vi "Get ChildNode by ctrl.vi"(8 "error in (no error)":errorcluster caption="错误输入（无错误）", 10 "ctr*":refnum<vi>, 11 "Node*":refnum<data-value>) -> (0 "error out":errorcluster caption="错误输出", 2 "ChildNode*":refnum<data-value>)   [LabVIEW 2016, in "PanelDataNode.lvclass"]
uses:
  PanelDataNode.lvclass
  PanelObject/PanelObject.lvclass
  C:/Users/CL/Desktop/ZcDAQprj0811/ZcDAQprj/Modules/DAQ-Display/PanelSplitToolkit/PanelLinkNode/PanelLinkNode.lvclass
  PanelLinkNode/PanelLinkNode.lvclass/PanelLinkNode.ctl
  PanelLinkNode/PanelLinkNode.lvclass
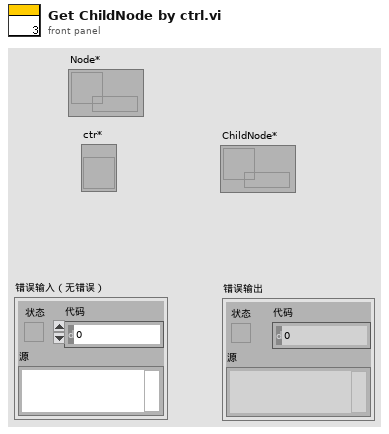
[diagram p1: front panel]
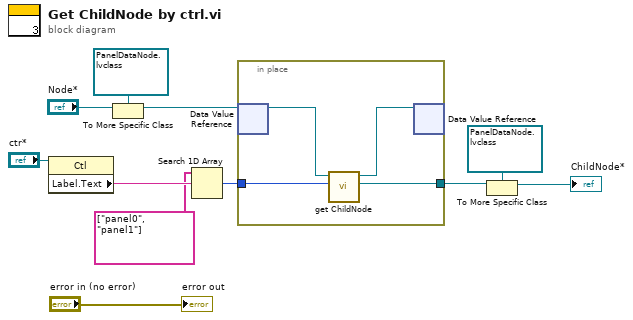
[diagram p0: block diagram]
diagram:
  n1 = property class="Ctl"(reference="ctr*") -> ("Label.Text"=w9:string)  [unwired: 1 in, 2 out]
  n2 = To More Specific Class(target class=refnum<data-value> refnum ("Node*"), reference="Node*") -> (specific class reference=w6:refnum<data-value>)  [unwired: 1 in, 1 out]
  n3 = Search 1D Array(1D array=string[] ["panel0", "panel1"], element=w9) -> (index of element=w7:i32)  [unwired: 1 in]
  n4 = in-place {
    in-place-border: w7 -> [w15]
    in-place-border: [w12] -> w3
    n5 = in-place-dvr #1(w6) -> (w14:refnum<class "PanelDataNode.lvclass">)  [unwired: 1 out]
    n6 = call "get ChildNode.vi"("index"=w15, "PanelLinkNode输入"=w14) -> ("ChildNode*"=w12:refnum<data-value>, "PanelLinkNode输出"=w13:refnum<class "PanelDataNode.lvclass">)  [unwired: 7 in, 1 out]
    n7 = in-place-dvr #1(w13) -> ()  [unwired: 2 out]
  }
  n8 = To More Specific Class(target class=refnum<data-value> refnum ("Node*"), reference=w3) -> (specific class reference=→"ChildNode*":refnum<data-value>)  [unwired: 1 in, 1 out]
  "error out" <- "error in (no error)"
